vi "ARGB Image Global.vi"() -> ()   [LabVIEW 2025]
uses:
  <vilib>/Serenial/G Augmented-Reality Toolkit/g_ar_toolkit.image/ARGB Image.ctl
  <vilib>/Serenial/G Augmented-Reality Toolkit/g_ar_toolkit.image/g_ar_toolkit.image.lvlib
panel:
  out "ARGB Image":T1
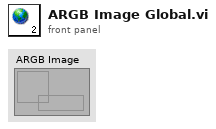
[diagram p1: front panel]
types:
  T1 = typedef "g_ar_toolkit.image.lvlib/ARGB Image.ctl" = refnum<data-value>
diagram:
